vi "Menu_Cluster Terminal.vi"(11 "Affected Items":T1) -> (3 "Menu Items To Add":T2(array[cluster]))   [LabVIEW 2023]
uses:
  top/BundleMagic.ctl
  controls/action enum.ctl
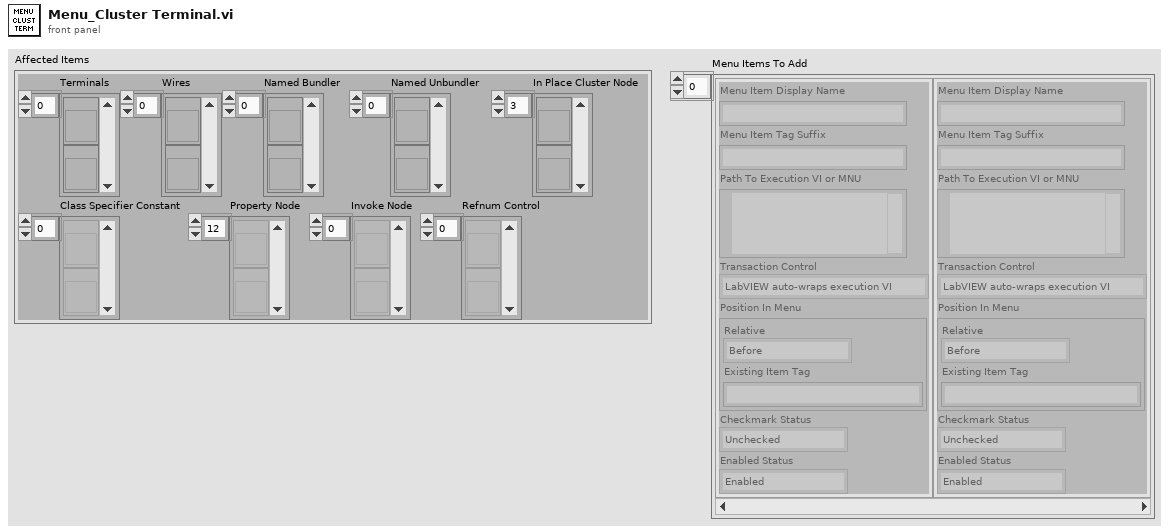
[diagram p1: front panel]
types:
  T1 = typedef "BundleMagic.ctl" = cluster{"Terminals":refnum<vi>[], "Wires":refnum<vi>[], "Named Bundler":refnum<vi>[], "Named Unbundler":refnum<vi>[], "In Place Cluster Node":refnum<vi>[], "Class Specifier Constant":refnum<vi>[], "Property Node":refnum<vi>[], "Invoke Node":refnum<vi>[], "Refnum Control":refnum<vi>[]}
  T2 = cluster{"Menu Item Display Name":string, "Menu Item Tag Suffix":string, "Path To Execution VI or MNU":path, "Transaction Control":enum8{"LabVIEW auto-wraps execution VI", "Execution VI will define if needed"}, "Position In Menu":cluster{"Relative":enum8{"Before", "Instead of", "After", "Into Submenu"}, "Existing Item Tag":string}, "Checkmark Status":enum8{"Unchecked", "Checked"}, "Enabled Status":enum8{"Enabled", "Disabled"}}[]
  T3 = typedef "action enum.ctl" = enum16{"[NONE]", "APP_SEPARATOR", "Wire Bundle", "Wire Unbundle", "Terminal Unbundle", "Terminal Bundle", "Bundler Move Up", "Bundler Move Down", "Bundler Insert", "Bundler Remove", "Bundler Remove Unwired", "Bundler Rearrange", "In Place Insert", "In Place Remove", "In Place Remove Unwired", "In Place Rearrange", "Wire Properties", "Wire Method", "Terminal Properties", "Terminal Method", "Property Move Up", "Property Move Down", "Properties Insert", "Properties Remove", "Properties Remove Unwired", "Properties Rearrange", "Method Change", "Class For Constant", "Class For Control", "Class For Node", "Class Name to Clipboard"}
  T4 = cluster{"Relative":enum8{"Before", "Instead of", "After", "Into Submenu"}, "Existing Item Tag":string}
  T5 = cluster{"Relative":enum8{"Before", "Instead of", "After", "Into Submenu"}, "Existing Item Tag":string}[]
  T6 = cluster{"Menu Item Display Name":string, "Menu Item Tag Suffix":string, "Path To Execution VI or MNU":path, "Transaction Control":enum8{"LabVIEW auto-wraps execution VI", "Execution VI will define if needed"}, "Position In Menu":cluster{"Relative":enum8{"Before", "Instead of", "After", "Into Submenu"}, "Existing Item Tag":string}, "Checkmark Status":enum8{"Unchecked", "Checked"}, "Enabled Status":enum8{"Enabled", "Disabled"}}
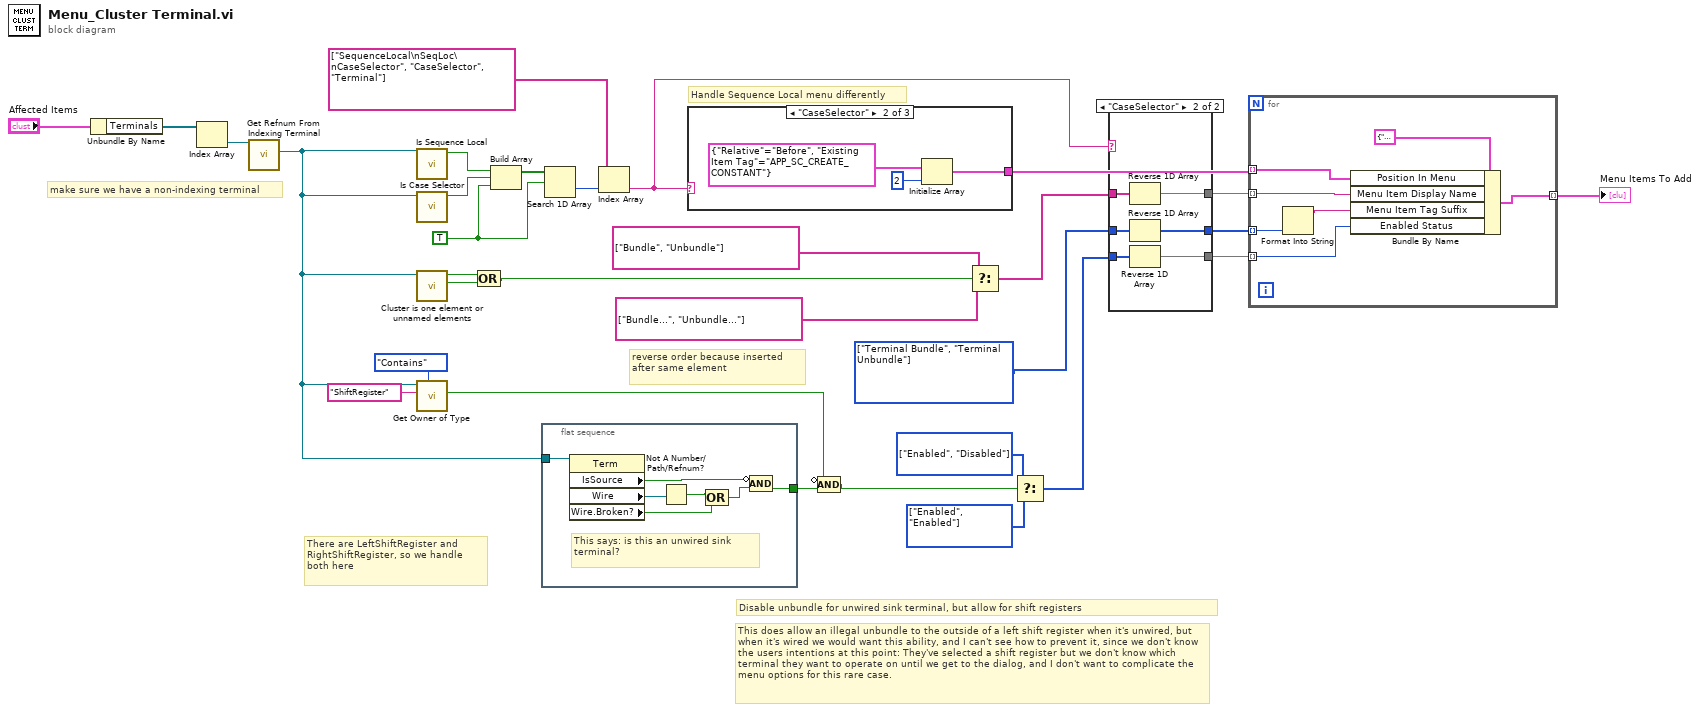
[diagram p0: block diagram]
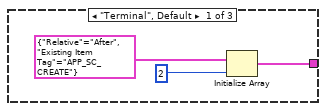
[diagram p3: hidden frame]
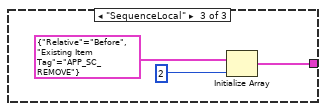
[diagram p4: hidden frame]
diagram:
  w1 = T3[] [enum."Terminal Bundle", enum."Terminal Unbundle"] items=["[NONE]", "APP_SEPARATOR", "Wire Bundle", "Wire Unbundle", "Terminal Unbundle", "Terminal Bundle", "Bundler Move Up", "Bundler Move Down", "Bundler Insert", "Bundler Remove", "Bundler Remove Unwired", "Bundler Rearrange", "In Place Insert", "In Place Remove", "In Place Remove Unwired", "In Place Rearrange", "Wire Properties", "Wire Method", "Terminal Properties", "Terminal Method", "Property Move Up", "Property Move Down", "Properties Insert", "Properties Remove", "Properties Remove Unwired", "Properties Rearrange", "Method Change", "Class For Constant", "Class For Control", "Class For Node", "Class Name to Clipboard"] ("Array")
  w9 = TRUE
  w28 = enum8{"Enabled", "Disabled"}[] [enum."Enabled", enum."Enabled"] items=["Enabled", "Disabled"] ("Enabled Status")
  w27 = enum8{"Enabled", "Disabled"}[] [enum."Enabled", enum."Disabled"] items=["Enabled", "Disabled"] ("Enabled Status")
  # "make sure we have a non-indexing terminal"
  # "There are LeftShiftRegister and RightShiftRegister, so we handle both here"
  # "This does allow an illegal unbundle to the outside of a left shift register when it's unwired, but when it's wired we would want this ability, and I can't see how to prevent it, since we don't know the users intentions at this point: They've selected a shift register but we don't know which terminal they want to operate on until we get to the dialog, and I don't want to complicate the menu options for this rare case."
  # "reverse order because inserted after same element"
  # "Disable unbundle for unwired sink terminal, but allow for shift registers"
  # "Handle Sequence Local menu differently"
  n1 = Unbundle By Name("Affected Items") -> ("Terminals"=w29:refnum<vi>[])
  n2 = Index Array(array=w29) -> (element=w15:refnum<vi>)  [unwired: 1 in]
  n3 = call "Get Refnum From Indexing Terminal.vi"("Refnum Terminal"=w15) -> ("Chosen Terminal"=w11:refnum<vi>)  [unwired: 8 in, 2 out]
  n4 = call "Is Sequence Local.vi"("Terminal in"=w11) -> ("Is Seq Local?"=w6:bool)  [unwired: 9 in, 1 out]
  n5 = call "Is Case Selector.vi"("Terminal in"=w11) -> ("Is Case Selector"=w12:bool)  [unwired: 9 in, 1 out]
  n6 = call "Cluster is one element or unnamed elements.vi"("Cluster Terminal"=w11) -> ("All Unnamed?"=w16:bool, "One Element?"=w17:bool)  [unwired: 8 in, 1 out]
  n7 = call "Get Owner of Type.vi"("Match Type"=enum16{"Exact Match", "Contains"}."Contains", "Owner Class Name desired"="ShiftRegister", "reference"=w11) -> ("Owner of type found?"=w21:bool)  [unwired: 4 in, 4 out]
  n8 = Compound Arithmetic op=OR(w17, w16) -> (w14:bool)
  n9 = Build Array(w6, w12, w9) -> (w10:bool[])
  n10 = flat-sequence {
    tunnel: [w34] -> w23
    tunnel: w11 -> [w33]
    frame #0 {
      # "This says: is this an unwired sink terminal?"
      n11 = property class="Term"(reference=w33) -> ("IsSource"=w32:bool, "Wire"=w38:refnum<vi>, "Wire.Broken?"=w36:bool)  [unwired: 1 in, 2 out]
      n12 = Not A Number/Path/Refnum?(number/path/refnum=w38) -> (NaN/Path/Refnum?=w37:bool)
      n13 = Compound Arithmetic op=OR(w37, w36) -> (w35:bool)
      n14 = Compound Arithmetic op=AND(invert w32, w35) -> (w34:bool)
    }
  }
  n15 = Search 1D Array(1D array=w10, element=w9) -> (index of element=w7:i32)  [unwired: 1 in]
  n16 = Index Array(array=string[] ["SequenceLocal\nSeqLoc\nCaseSelector", "CaseSelector", "Terminal"], index=w7) -> (element=w2:string)
  n17 = case shown="\"CaseSelector\"" w2 {
    tunnel: [w39 w42 w45] -> w30
    frame "Terminal", Default {
      n18 = Initialize Array(T4 {"Relative"=enum."After", "Existing Item Tag"="APP_SC_CREATE"} ("Position In Menu"), 2) -> (w39:T5)
    }
    frame "CaseSelector" {
      n19 = Initialize Array(T4 {"Relative"=enum."Before", "Existing Item Tag"="APP_SC_CREATE_CONSTANT"} ("Position In Menu"), 2) -> (w42:T5)
    }
    frame "SequenceLocal" {
      n20 = Initialize Array(T4 {"Relative"=enum."Before", "Existing Item Tag"="APP_SC_REMOVE"} ("Position In Menu"), 2) -> (w45:T5)
    }
  }
  n21 = Compound Arithmetic op=AND(invert w21, w23) -> (w22:bool)
  n22 = Select(t=string[] ["Bundle", "Unbundle"], s=w14, f=string[] ["Bundle...", "Unbundle..."]) -> (s? t:f=w18:string[])
  n23 = Select(t=w27, s=w22, f=w28) -> (s? t:f=w26:enum8{"Enabled", "Disabled"}[])
  n24 = case shown="\"CaseSelector\"" w2 {
    tunnel: w26 -> [w48 w56]
    tunnel: w1 -> [w49 w55]
    tunnel: w18 -> [w50 w54]
    tunnel: [w50 w53] -> w5
    tunnel: [w49 w52] -> w4
    tunnel: [w48 w51] -> w3
    frame Default {
    }
    frame "CaseSelector" {
      n25 = Reverse 1D Array(array=w54) -> (reversed array=w53:string[])
      n26 = Reverse 1D Array(array=w55) -> (reversed array=w52:T3[])
      n27 = Reverse 1D Array(array=w56) -> (reversed array=w51:enum8{"Enabled", "Disabled"}[])
    }
  }
  n28 = for {
    tunnel: [w61] -> w31 mode=indexing
    tunnel: w30 -> [w59] mode=indexing
    tunnel: w5 -> [w62] mode=indexing
    tunnel: w3 -> [w60] mode=indexing
    tunnel: w4 -> [w57] mode=indexing
    n29 = Format Into String(w57) -> (resulting string=w58:string)  [unwired: 3 in, 1 out]
    n30 = Bundle By Name(cluster=T6 {"Menu Item Display Name"="", "Menu Item Tag Suffix"="", "Path To Execution VI or MNU"=path "", "Transaction Control"=enum."LabVIEW auto-wraps execution VI", "Position In Menu"={"Relative"=enum."Before", "Existing Item Tag"=""}, "Checkmark Status"=enum."Unchecked", "Enabled Status"=enum."Enabled"} ("Cluster"), "Position In Menu"=w59, "Menu Item Display Name"=w62, "Menu Item Tag Suffix"=w58, "Enabled Status"=w60) -> (w61:T6)
  }
  "Menu Items To Add" <- w31
